vi "WriteI32ClusterArray.vi"(8 "ErrorIn(No Error)":errorcluster caption="entrée d'erreur (pas d'erreur)", 9 "Data":i32=-1, 10 "array":cluster{"Tableau":i32[]}[](array[cluster]), 11 "ClusterInd":i32=-1) -> (0 "sortie d'erreur":errorcluster, 2 "output array":cluster{"Tableau":i32[]}[](array[cluster]))   [LabVIEW 2019]
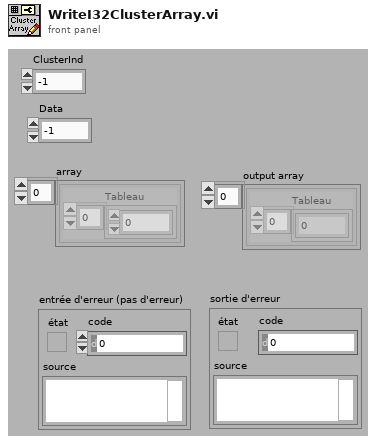
[diagram p1: front panel]
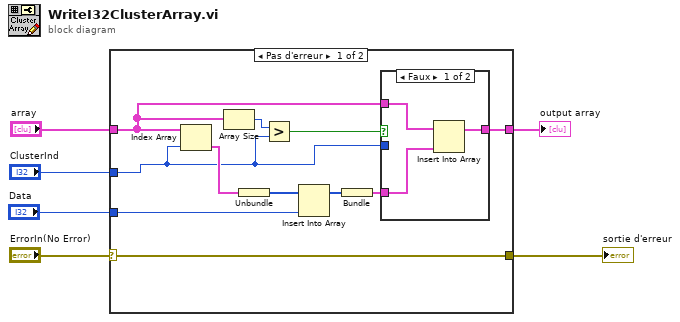
[diagram p0: block diagram]
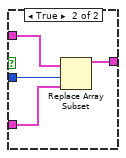
[diagram p2: hidden frame]
diagram:
  n1 = case shown="Pas d'erreur" "ErrorIn(No Error)" {
    selector: "ErrorIn(No Error)" -> [w16 w26]
    tunnel: [w16 w26] -> w5
    tunnel: "Data" -> [w17 _]
    tunnel: "ClusterInd" -> [w8 _]
    tunnel: "array" -> [w10 w25]
    tunnel: [w15 w25] -> w1
    frame No Error {
      n2 = Index Array(array=w10, index=w8) -> (element=w12:cluster{"Tableau":i32[]})
      n3 = Array Size(array=w10) -> (size(s)=w9:i32)
      n4 = Unbundle(w12) -> ("Tableau"=w14:i32[])
      n5 = Greater?(x=w9, y=w8) -> (0:w7:bool)
      n6 = Insert Into Array(array=w14, new element=w17) -> (w13:i32[])  [unwired: 1 in]
      n7 = Bundle("Tableau"=w13) -> (w11:cluster{"Tableau":i32[]})  [unwired: 1 in]
      n8 = case shown="Faux" w7 {
        tunnel: w10 -> [w20 w24]
        tunnel: [w19 w23] -> w15
        tunnel: w8 -> [_ w22]
        tunnel: w11 -> [w18 w21]
        frame False {
          n9 = Insert Into Array(array=w20, new element=w18) -> (w19:cluster{"Tableau":i32[]}[])  [unwired: 1 in]
        }
        frame True {
          n10 = Replace Array Subset(array=w24, new element=w21, index=w22) -> (w23:cluster{"Tableau":i32[]}[])
        }
      }
    }
    frame Error {
    }
  }
  "sortie d'erreur" <- w5
  "output array" <- w1
